vi "RichToFlatgoogle_protobuf_Option.vi"(5 "OutputClusterType":T1, 11 "InputCluster":T3) -> (3 "OutputCluster":T1)   [LabVIEW 2020, in "Measurement Plugin Measurement Service Base V2.lvlib"]
uses:
  Measurement Plugin Measurement Service Base V2.lvlib
  google_protobuf_Option.ctl
  google_protobuf_Any.ctl
  google_protobuf_Option_Flat.ctl
  google_protobuf_Any_Flat.ctl
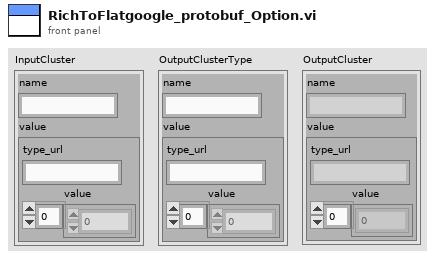
[diagram p1: front panel]
types:
  T1 = typedef "Measurement Plugin Measurement Service Base V2.lvlib/google_protobuf_Option_Flat.ctl" = cluster{"name":string, "value":T2}
  T2 = typedef "Measurement Plugin Measurement Service Base V2.lvlib/google_protobuf_Any_Flat.ctl" = cluster{"type_url":string, "value":u8[]}
  T3 = typedef "Measurement Plugin Measurement Service Base V2.lvlib/google_protobuf_Option.ctl" = cluster{"name":string, "value":T4}
  T4 = typedef "Measurement Plugin Measurement Service Base V2.lvlib/google_protobuf_Any.ctl" = cluster{"type_url":string, "value":u8[]}
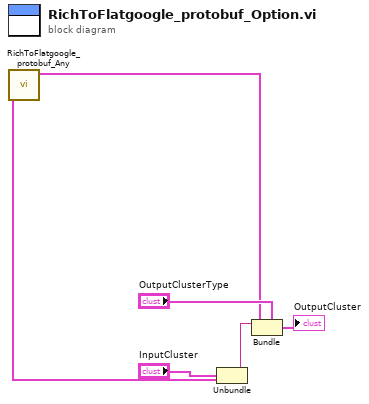
[diagram p0: block diagram]
diagram:
  n1 = Unbundle "Unbundle"("InputCluster") -> ("name"=w3:string, "value"=w2:T4)
  n2 = call "RichToFlatgoogle_protobuf_Any.vi"("InputCluster"=w2) -> ("OutputCluster"=w1:T2)  [unwired: 10 in]
  n3 = Bundle "Bundle"(cluster="OutputClusterType", "name"=w3, "value"=w1) -> (→"OutputCluster":T1)
